vi "Top Level.vi"   [LabVIEW 2014]
uses:
  Global Booleans Enum.ctl
types:
  T1 = typedef "Global Booleans Enum.ctl" = enum16{"all stop", "Play", "Image Aligned?"}
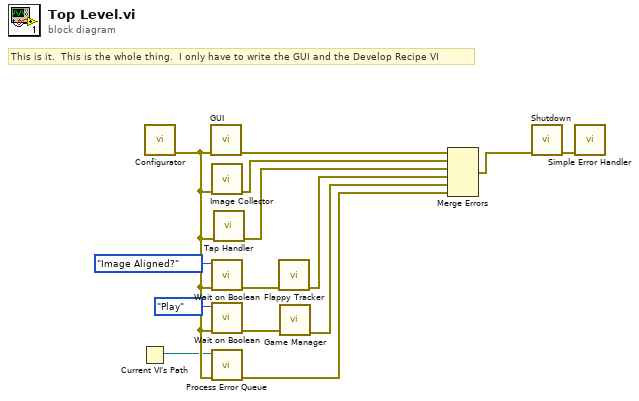
[diagram p0: block diagram]
diagram:
  # "This is it.  This is the whole thing.  I only have to write the GUI and the Develop Recipe VI"
  n1 = Current VI's Path() -> (path=w1:path)
  n2 = call "Configurator.vi"() -> ("error out"=w3:errorcluster)  [unwired: 11 in]
  n3 = call "GUI.vi"("error in (no error)"=w3) -> ("error out"=w9:errorcluster)  [unwired: 10 in]
  n4 = call "Image Collector.vi"("error in (no error)"=w3) -> ("error out"=w10:errorcluster)  [unwired: 10 in]
  n5 = call "Wait on Boolean.vi"("error in (no error)"=w3, "Global boolean to wait on"=Global_Booleans_Enum."Image Aligned?") -> ("error out"=w6:errorcluster)  [unwired: 9 in]
  n6 = call "Wait on Boolean.vi"("error in (no error)"=w3, "Global boolean to wait on"=Global_Booleans_Enum."Play") -> ("error out"=w7:errorcluster)  [unwired: 9 in]
  n7 = call "Process Error Queue.vi"("error in (no error)"=w3, "Base Path"=w1) -> ("error out"=w2:errorcluster)  [unwired: 9 in]
  n8 = call "Tap Handler.vi"("error in (no error)"=w3) -> ("error out"=w11:errorcluster)  [unwired: 10 in]
  n9 = call "Flappy Tracker.vi"("error in (no error)"=w6) -> ("error out"=w12:errorcluster)  [unwired: 10 in]
  n10 = call "Game Manager.vi"("error in (no error)"=w7) -> ("error out"=w8:errorcluster)  [unwired: 10 in]
  n11 = Merge Errors(w9, w10, w11, w12, w8, w2) -> (w13:errorcluster)
  n12 = call "Shutdown.vi"("error in (no error)"=w13) -> ("error out"=w14:errorcluster)  [unwired: 10 in]
  n13 = call <vilib>:"Simple Error Handler.vi"("error in (no error)"=w14) -> ()  [unwired: 4 in, 5 out]
